vi "YKMW100 Mode Control.vi"(0 "VISA session":refnum<visa-resource-name>="MW100", 5 "Model":enum16{"Meausurement Mode", "Setting Mode"}(ring), 11 "error in (no error)":errorcluster) -> (4 "dup VISA session":refnum<visa-resource-name>="MW100", 15 "error out":errorcluster)   [LabVIEW 2016]
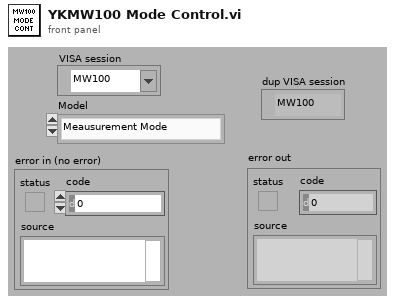
[diagram p1: front panel]
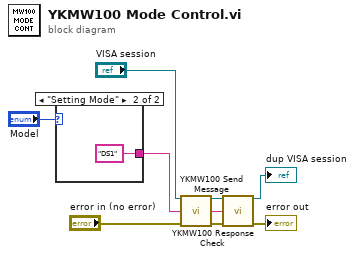
[diagram p0: block diagram]
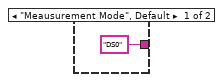
[diagram p2: hidden frame]
diagram:
  n1 = case shown="\"Setting Mode\"" "Model" {
    tunnel: ["DS0" ("Send Message (\"\")") "DS1" ("Send Message (\"\")")] -> w2
    frame "Meausurement Mode", Default {
    }
    frame "Setting Mode" {
    }
  }
  n2 = call "YKMW100 Send Message.vi"("VISA session"="VISA session", "Send Message (\"\")"=w2, "error in (no error)"="error in (no error)") -> ("dup VISA session"=w7:refnum<visa-resource-name>, "Read Buffer"=w5:string, "error out"=w6:errorcluster)  [unwired: 10 in]
  n3 = call "YKMW100 Response Check.vi"("VISA session"=w7, "Message In (\"\")"=w5, "error in (no error)"=w6) -> ("dup VISA session"=→"dup VISA session":refnum<visa-resource-name>, "error out"=→"error out":errorcluster)  [unwired: 8 in, 3 out]
